vi "Determine User Targets.vi"(11 "Targets":enum16{"Linux_x64", "Windows", "All"}(ring)) -> (3 "User Configured Targets":enum16{"Linux_x64", "Windows", "All"}[](array[ring]))   [LabVIEW 2026, in "NIVS_CDEW_MetaDataObj.lvclass"]
uses:
  NIVS_CDEW_MetaDataObj.lvclass
  NIVS_CDEW_MetaDataObj.lvclass/NIVS_CDEW_MetaDataObj.ctl
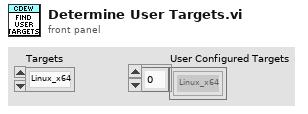
[diagram p1: front panel]
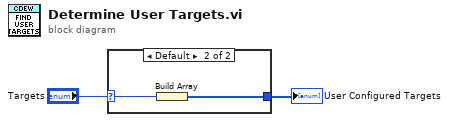
[diagram p0: block diagram]
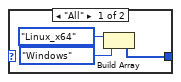
[diagram p2: hidden frame]
diagram:
  n1 = case shown="Default" "Targets" {
    selector: "Targets" -> [_ w7]
    tunnel: [w3 w6] -> w1
    frame "All" {
      n2 = Build Array(enum16{"Linux_x64", "Windows", "All"}."Linux_x64" ("Target Types"), enum16{"Linux_x64", "Windows", "All"}."Windows" ("Target Types")) -> (w3:enum16{"Linux_x64", "Windows", "All"}[])
    }
    frame Default {
      n3 = Build Array(w7) -> (w6:enum16{"Linux_x64", "Windows", "All"}[])
    }
  }
  "User Configured Targets" <- w1
